vi "Receive - Monitor.vi"() -> ()   [LabVIEW 2020]
uses:
  <instrlib>/AIM GmbH/_AIM 664/_controls/session_monitor_config.ctl
  <instrlib>/AIM GmbH/_AIM 664/_controls/monitor_becw_type.ctl
  <instrlib>/AIM GmbH/_AIM 664/_controls/monitor_fhInfol_type.ctl
  <instrlib>/AIM GmbH/_AIM 664/_controls/monitor_entrySize_type.ctl
  <instrlib>/AIM GmbH/_AIM 664/_controls/monitor_fhw0_type.ctl
  <instrlib>/AIM GmbH/_AIM 664/_controls/monitor_fhw1_type.ctl
  <instrlib>/AIM GmbH/_AIM 664/_polimorphicInstances/session/CreateSession(RX-Monitor).vi
  <instrlib>/AIM GmbH/_AIM 664/_polimorphicInstances/control/Start (Rx).vi
  <instrlib>/AIM GmbH/_AIM 664/_polimorphicInstances/control/Stop (Rx).vi
  <instrlib>/AIM GmbH/_AIM 664/_polimorphicInstances/session/CleanupSession (Port).vi
  <instrlib>/AIM GmbH/_AIM 664/AIM664LV.lvlib
panel:
  out "IrigTime":T1
  out "FrameHeaderInfo":T2 {"FHW0"."MacID" format="%03b"}
  out "BECW":T6
  out "Payload":u8[](array[numeric]) format="%.0x"
  out "Synchronized":u32
  in  "EntryCount (1)":u32=1
  out "QueueStatus":T7 {"QueueStatus" items=["FDX_MON_STAT_EMPTY", "FDX_MON_STAT_ FILLED", "FDX_MON_STAT_ FULL", "FDX_MON_STAT_ OVERFLOW", "FDX_MON_STAT_ ERROR"]}
  out "Curent Irig Time":T8
  in  "fetch period ms":u32=100
  in  "MaxFileSize MB (1)":u32=1
  in  "MonCapMode":T9 {"Strobe" items=["FDX_MON_STROBE_DIS", "FDX_MON_STROBE_STOP", "FDX_MON_STROBE_START"]; "CaptureMode" items=["FDX_MON_SINGLE ", "FDX_MON_CONTINUOUS", "FDX_MON_SELECTIVE", "FDX_MON_RECORDING", "FDX_MON_REROS", "FDX_MON_HMU"]}
  out "PortInitOut":T10 {"PortConfig" items=["FDX_SINGLE", "FDX_REDUNDANT"]}
  in  "port":u32=1
  in  "board":u32
  in  "MonitorConfig":T11={"DefaultCronoMode"=2, "GlbMonBufferSizeIn"=0} {"DefaultCronoMode" items=["FDX_RX_DEFAULT_ENA_CNT", "FDX_RX_DEFAULT_MON_ENA_ALL", "FDX_RX_DEFAULT_MON_ENA_GOOD"]}
  out "error out":errorcluster
  in  "stop":bool
  out "current time":timestamp
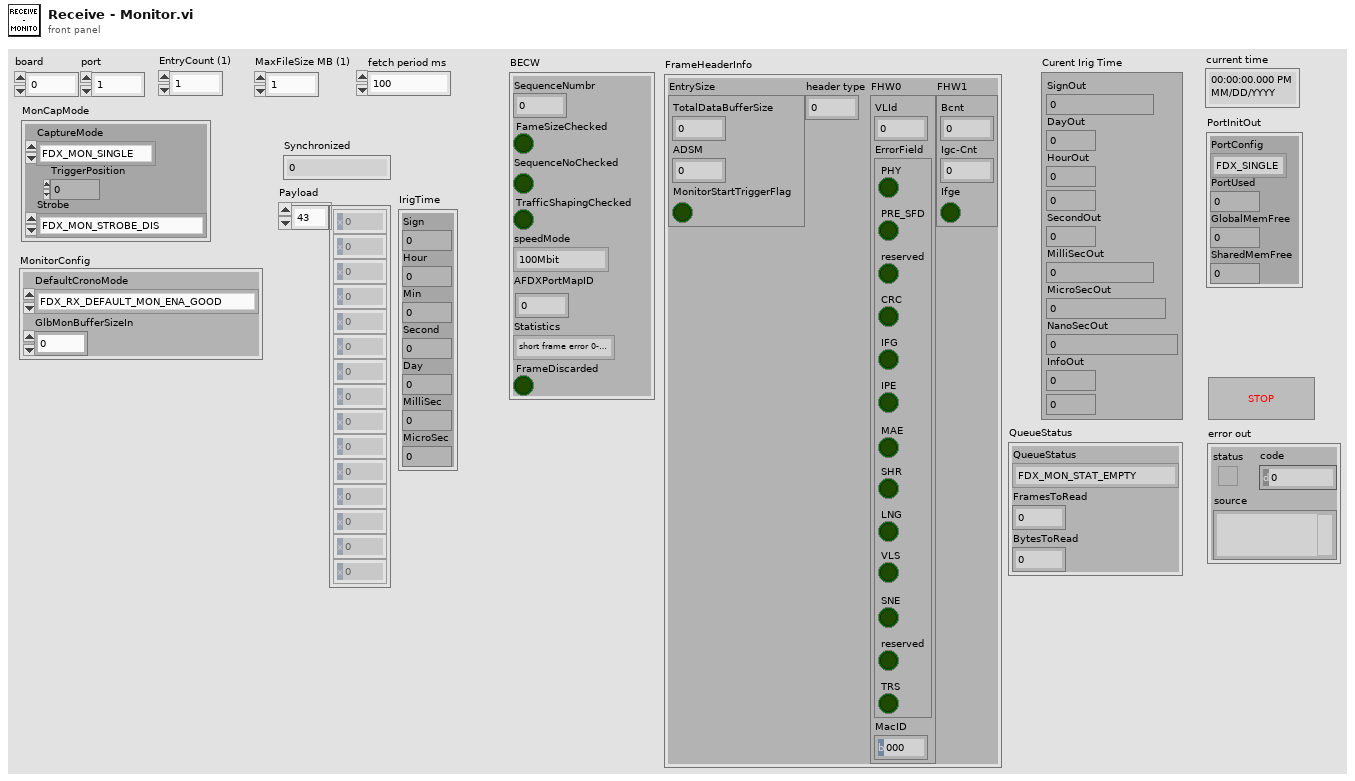
[diagram p1: front panel]
types:
  T1 = cluster{"Sign":i32, "Hour":u32, "Min":u32, "Second":u32, "Day":u32, "MilliSec":u32, "MicroSec":u32}
  T2 = typedef "AIM664LV.lvlib/monitor_fhInfol_type.ctl" = cluster{"EntrySize":T3, "header type":u32, "FHW0":T4, "FHW1":T5}
  T3 = typedef "AIM664LV.lvlib/monitor_entrySize_type.ctl" = cluster{"TotalDataBufferSize":u16, "ADSM":u16, "MonitorStartTriggerFlag":bool}
  T4 = typedef "AIM664LV.lvlib/monitor_fhw0_type.ctl" = cluster{"VLId":u16, "ErrorField":cluster{"PHY":bool, "PRE_SFD":bool, "reserved":bool, "CRC":bool, "IFG":bool, "IPE":bool, "MAE":bool, "SHR":bool, "LNG":bool, "VLS":bool, "SNE":bool, "reserved":bool, "TRS":bool}, "MacID":u8}
  T5 = typedef "AIM664LV.lvlib/monitor_fhw1_type.ctl" = cluster{"Bcnt":u16, "Igc-Cnt":u16, "Ifge":bool}
  T6 = typedef "AIM664LV.lvlib/monitor_becw_type.ctl" = cluster{"SequenceNumbr":u8, "FameSizeChecked":bool, "SequenceNoChecked":bool, "TrafficShapingChecked":bool, "speedMode":enum16{"100Mbit", "10Mbit", "1Gbit"}, "AFDXPortMapID":u8, "Statistics":enum16{"short frame error 0-63Bytes", "64-127 Bytes", "128-255 Bytes", "256-511 Bytes", "512-1023 Bytes", "1024-1518 Bytes", ">1518 Bytes"}, "FrameDiscarded":bool}
  T7 = cluster{"QueueStatus":u32, "FramesToRead":u32, "BytesToRead":u32}
  T8 = cluster{"SignOut":i32, "DayOut":u32, "HourOut":u32, "MinOut":u32, "SecondOut":u32, "MilliSecOut":u32, "MicroSecOut":u32, "NanoSecOut":u32, "InfoOut":u32, "Mode":u32}
  T9 = cluster{"CaptureMode":u32, "TriggerPosition":u32, "Strobe":u32}
  T10 = cluster{"PortConfig":u32, "PortUsed":u32, "GlobalMemFree":u32, "SharedMemFree":u32}
  T11 = typedef "AIM664LV.lvlib/session_monitor_config.ctl" = cluster{"DefaultCronoMode":u32, "GlbMonBufferSizeIn":u32}
  T12 = cluster{"EntryRead":u32, "BytesRead":u32, "Synchronized":u32, "ReadBuffer":u8[]}
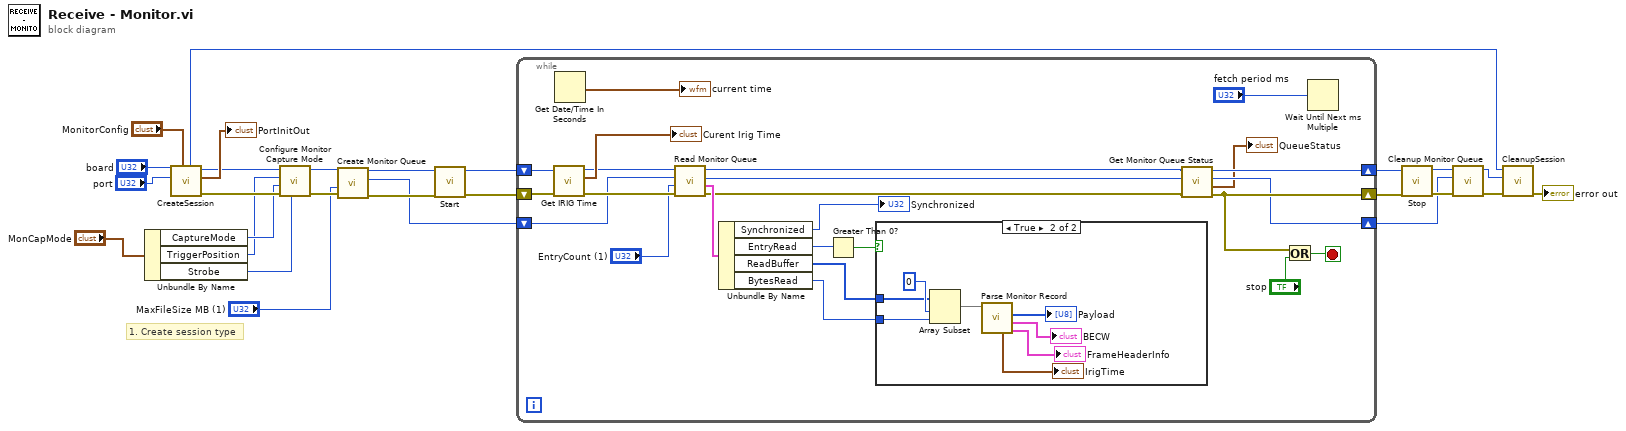
[diagram p0: block diagram]
diagram:
  # "1. Create session type"
  n1 = Unbundle By Name("MonCapMode") -> ("CaptureMode"=w6:u32, "TriggerPosition"=w5:u32, "Strobe"=w4:u32)
  n2 = call-poly <instrlib>:"CreateSession.vi"("MonitorConfig"="MonitorConfig", "port"="port", "board"="board") -> ("error out"=w17:errorcluster, "PortInitOut"=→"PortInitOut":T10, "InstrumentHandle_port out"=w18:u32, "InstrumentHandle_board out"=w9:u32)  [unwired: 3 in, 2 out]
  n3 = call <instrlib>:"Configure Monitor Capture Mode.vi"("Strobe"=w4, "error in (no error)"=w17, "CaptureMode"=w6, "TriggerPosition"=w5, "InstrumentHandle_port in"=w18) -> ("error out"=w16:errorcluster, "InstrumentHandle_port out"=w15:u32)  [unwired: 5 in]
  n4 = call <instrlib>:"Create Monitor Queue.vi"("error in (no error)"=w16, "MaxFileSize MB (1)"="MaxFileSize MB (1)", "InstrumentHandle_port in"=w15) -> ("error out"=w13:errorcluster, "QueueIdOut"=w12:u32, "InstrumentHandle_port out"=w14:u32)  [unwired: 5 in, 1 out]
  n5 = call-poly <instrlib>:"Start.vi"("error in (no error)"=w13, "InstrumentHandle_port in"=w14) -> ("error out"=w25:errorcluster, "InstrumentHandle_port out"=w27:u32)  [unwired: 8 in]
  n6 = while {
    shift-right: [w31] -> w26
    shift-left: w27 -> [w48]
    shift-right: [w35] -> w24
    shift-left: w25 -> [w47]
    shift-right: [w30] -> w1
    shift-left: w12 -> [w32]
    stop <- w49 stop-if-true
    n7 = call <instrlib>:"Get IRIG Time.vi"("error in (no error)"=w47, "InstrumentHandle_board in"=w48) -> ("error out"=w44:errorcluster, "Curent Irig Time"=→"Curent Irig Time":T8, "InstrumentHandle_board out"=w33:u32)  [unwired: 7 in]
    n8 = Get Date/Time In Seconds() -> (seconds since 1Jan1904=→"current time":timestamp)
    n9 = call <instrlib>:"Read Monitor Queue.vi"("error in (no error)"=w44, "EntryCount (1)"="EntryCount (1)", "QueueId in"=w32, "InstrumentHandle_port in"=w33) -> ("error out"=w36:errorcluster, "QueueReadOut"=w42:T12, "QueueId out"=w28:u32, "InstrumentHandle_port out"=w37:u32)  [unwired: 4 in]
    n10 = Unbundle By Name(w42) -> ("Synchronized"=→"Synchronized":u32, "EntryRead"=w41:u32, "ReadBuffer"=w39:u8[], "BytesRead"=w38:u32)
    n11 = Greater Than 0?(x=w41) -> (x > 0?=w43:bool)
    n12 = case shown="True" w43 {
      tunnel: w39 -> [_ w54]
      tunnel: w38 -> [_ w53]
      frame False {
      }
      frame True {
        n13 = Array Subset(array=w54, index=0, length=w53) -> (w52:u8[])
        n14 = call <instrlib>:"Parse Monitor Record.vi"("Record In"=w52) -> ("FrameHeaderInfo"=→"FrameHeaderInfo":T2, "BECW"=→"BECW":T6, "Payload"=→"Payload":u8[], "IrigTime"=→"IrigTime":T1)  [unwired: 5 in, 2 out]
      }
    }
    n15 = call <instrlib>:"Get Monitor Queue Status.vi"("error in (no error)"=w36, "QueueId in"=w28, "InstrumentHandle_port in"=w37) -> ("error out"=w35:errorcluster, "QueueStatus"=→"QueueStatus":T7, "QueueId out"=w30:u32, "InstrumentHandle_port out"=w31:u32)  [unwired: 5 in]
    n16 = Or(x=w35, y="stop") -> (x .or. y?=w49:bool)
    n17 = Wait Until Next ms Multiple(millisecond multiple="fetch period ms") -> ()  [unwired: 1 out]
  }
  n18 = call-poly <instrlib>:"Stop.vi"("error in (no error)"=w24, "InstrumentHandle_port in"=w26) -> ("error out"=w11:errorcluster, "InstrumentHandle_port out"=w3:u32)  [unwired: 8 in]
  n19 = call <instrlib>:"Cleanup Monitor Queue.vi"("error in (no error)"=w11, "QueueId"=w1, "InstrumentHandle_port in"=w3) -> ("error out"=w10:errorcluster, "InstrumentHandle_port out"=w2:u32)  [unwired: 7 in]
  n20 = call-poly <instrlib>:"CleanupSession.vi"("error in (no error)"=w10, "InstrumentHandle_port in"=w2, "InstrumentHandle_board in"=w9) -> ("error out"=→"error out":errorcluster)  [unwired: 8 in]
